vi "Get_Process_Details.vi"(0 "Process_Data":string[](array[string])) -> (4 "Needs":string[][](array[string]))   [LabVIEW 2023]
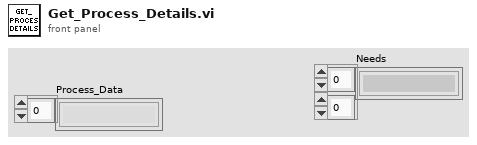
[diagram p1: front panel]
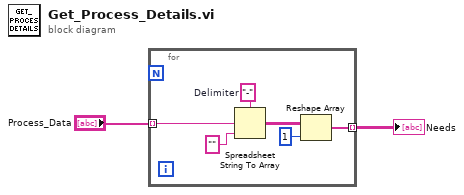
[diagram p0: block diagram]
diagram:
  n1 = for {
    tunnel: "Process_Data" -> [w8] mode=indexing
    tunnel: [w3] -> w1 mode=indexing
    w7 = "-"  # Delimiter
    n2 = Spreadsheet String To Array(delimiter (Tab)=w7, spreadsheet string=w8, array type (2D Dbl)="" ("format string")) -> (array=w5:string[][])  [unwired: 1 in]
    n3 = Reshape Array(w5, 1 ("dimension size")) -> (w3:string[])
  }
  "Needs" <- w1
